vi "Tree Checker.vi"() -> ()   [LabVIEW 2016]
panel:
  in  "Starting at N = ?":i32=2
  out "Finished?":bool
  out "Time By N":cluster{dbl, "Run Time ms":u32}[](graph)
  out "Radio Number By N":cluster{dbl, "Radio Number":i32}[](graph)
  out "Start Value by N":cluster{dbl, "Start Value":i32}[](graph)
  out "Total time Progressed":u32
  in  "Up to N = ?":i32
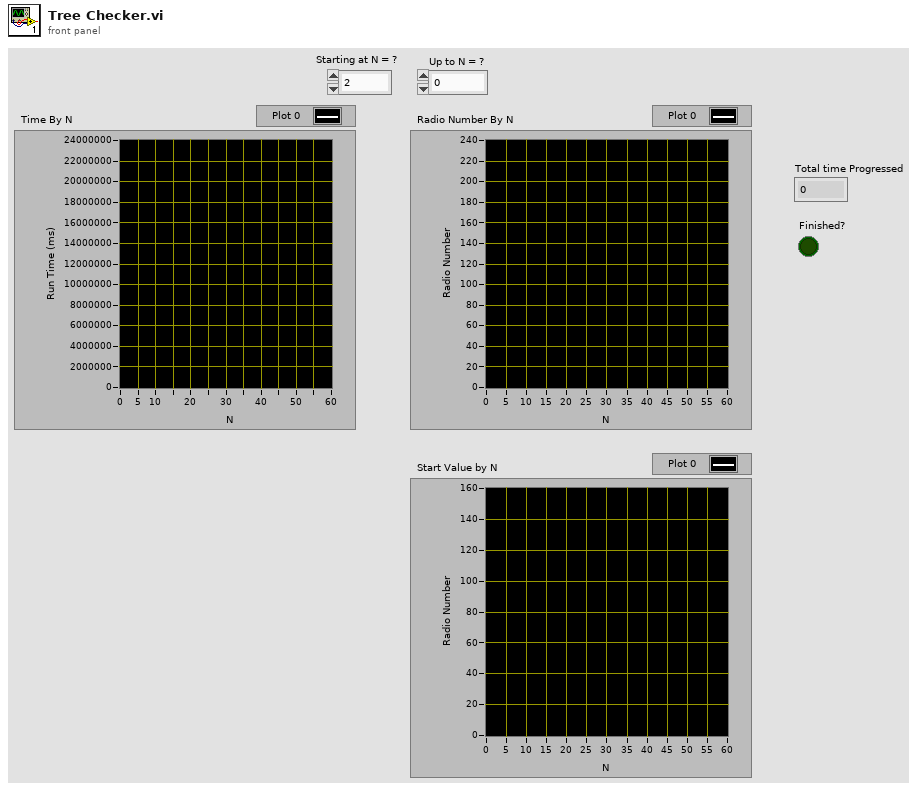
[diagram p1: front panel]
types:
  T1 = typedef "NI_Matrix.lvlib/RealMatrix.ctl" = dbl[][]
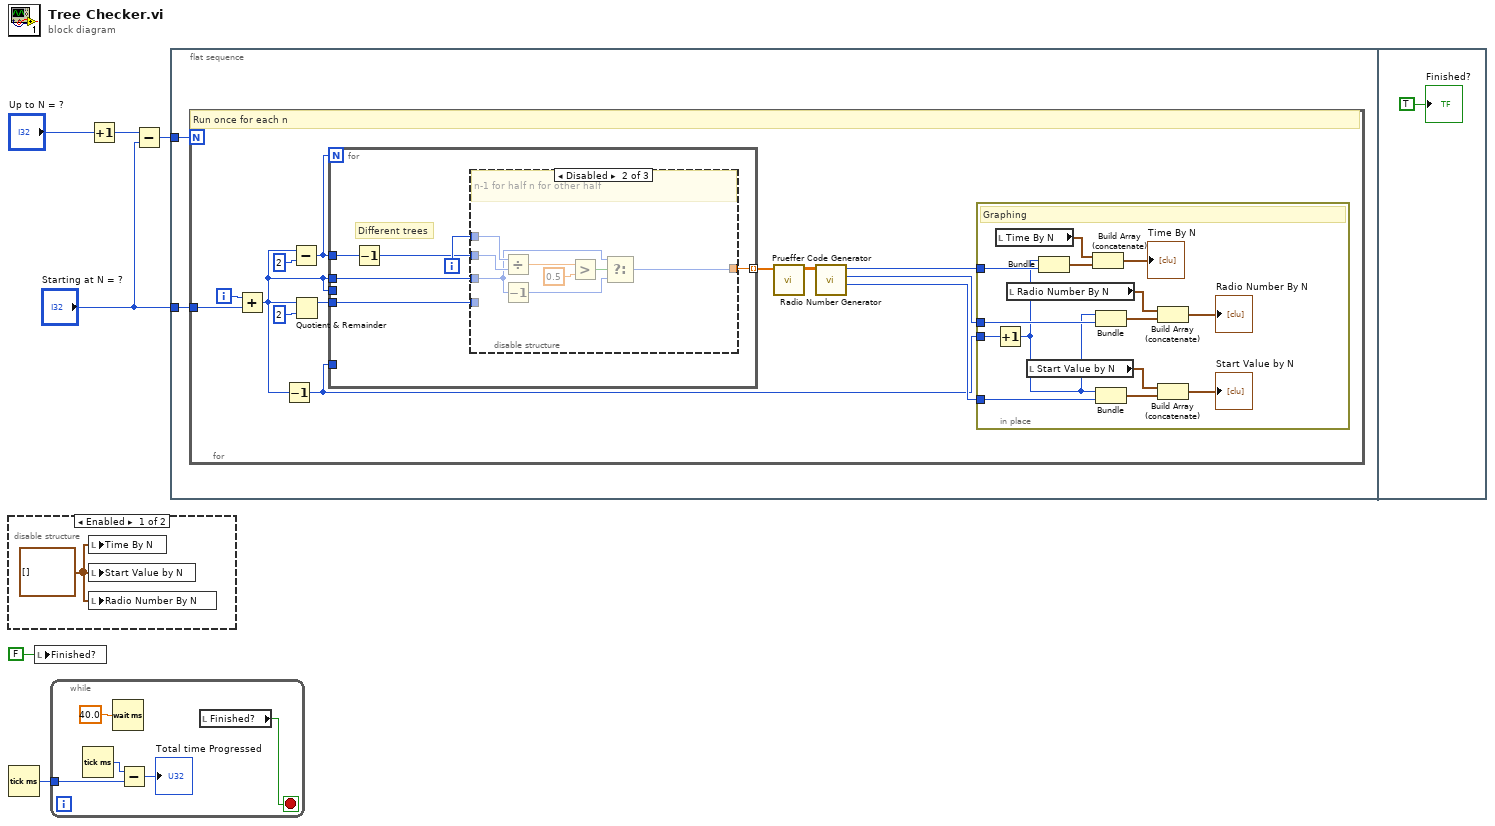
[diagram p0: block diagram]
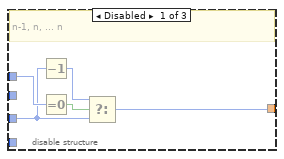
[diagram p2: hidden frame]
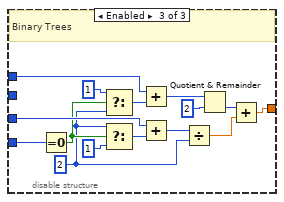
[diagram p3: hidden frame]
diagram:
  n1 = disable-structure shown="Enabled" {
    frame Enabled {
      w7 = cluster{i32, "Radio Number":i32}[] [] ("appended array")
      n2 = local write "Time By N"(w7) -> ()
      n3 = local write "Start Value by N"(w7) -> ()
      n4 = local write "Radio Number By N"(w7) -> ()
    }
    frame Disabled {
    }
  }
  n5 = Tick Count (ms)() -> (millisecond timer value=w4:u32)
  n6 = local write "Finished?"(FALSE) -> ()
  n7 = while {
    tunnel: w4 -> [w9]
    stop <- w11 stop-if-true
    n8 = Tick Count (ms)() -> (millisecond timer value=w10:u32)
    n9 = Wait (ms)(milliseconds to wait=40.0) -> ()  [unwired: 1 out]
    n10 = Subtract(x=w10, y=w9) -> (x-y=→"Total time Progressed":u32)
    n11 = local read "Finished?"() -> (w11:bool)
  }
  n12 = Increment(x="Up to N = ?") -> (x+1=w1:i32)
  n13 = Subtract(x=w1, y="Starting at N = ?") -> (x-y=w5:i32)
  n14 = flat-sequence {
    tunnel: w5 -> [w14]
    tunnel: "Starting at N = ?" -> [w13]
    frame #0 {
      n15 = for {
        N: w14 -> [_]
        tunnel: w13 -> [w24]
        i -> [w27]
        # "Run once for each n"
        n16 = Add(x=w27, y=w24) -> (x+y=w16:i32)
        n17 = Decrement(x=w16) -> (x-1=w19:i32)
        n18 = Subtract(x=w16, y=2) -> (x-y=w18:i32)
        n19 = Quotient & Remainder(x=w16, y=2) -> (x-y*floor(x/y)=w15:i32)  [unwired: 1 out]
        n20 = for {
          N: w18 -> [_]
          tunnel: w16 -> [_]
          tunnel: [w32] -> w22 mode=indexing
          tunnel: w19 -> [_]
          tunnel: w16 -> [w31]
          tunnel: w18 -> [w30]
          tunnel: w15 -> [w28]
          i -> [w33]
          # "Different trees"
          n21 = Decrement(x=w30) -> (x-1=w29:i32)
          n22 = disable-structure shown="Disabled" {
            disable-tunnel: w33 -> [w37 w46 w60]
            disable-tunnel: [w34 w45 w51] -> w32
            disable-tunnel: w31 -> [w36 w39 w55]
            disable-tunnel: w29 -> [_ w44 _]
            disable-tunnel: w28 -> [_ _ w57]
            frame Disabled {
              # "n-1, n, ... n"
              n23 = Decrement(x=w36) -> (x-1=w35:i32)
              n24 = Equal To 0?(x=w37) -> (x = 0?=w38:bool)
              n25 = Select(t=w35, s=w38, f=w36) -> (s? t:f=w34:i32)
            }
            frame Disabled {
              # "n-1 for half n for other half"
              n26 = Divide(x=w46, y=w44) -> (x/y=w43:dbl)
              n27 = Decrement(x=w39) -> (x-1=w40:i32)
              n28 = Greater?(x=w43, y=0.5) -> (0:w41:bool)
              n29 = Select(t=w39, s=w41, f=w40) -> (s? t:f=w45:i32)
            }
            frame Enabled {
              w48 = 2 ("f")
              # "Binary Trees"
              n30 = Equal To 0?(x=w57) -> (x = 0?=w49:bool)
              n31 = Select(t=1 ("y"), s=w49, f=w48) -> (s? t:f=w54:i32)
              n32 = Select(t=w48, s=w49, f=1 ("y")) -> (s? t:f=w47:i32)
              n33 = Add(x=w60, y=w54) -> (x+y=w59:i32)
              n34 = Add(x=w55, y=w47) -> (x+y=w53:i32)
              n35 = Divide(x=w53, y=w48) -> (x/y=w52:dbl)
              n36 = Quotient & Remainder(x=w59, y=2) -> (floor(x/y)=w58:i32)  [unwired: 1 out]
              n37 = Add(x=w58, y=w52) -> (x+y=w51:dbl)
            }
          }
        }
        n38 = call "Prueffer Code Generator.vi"("Array"=w22) -> ("Adjacency Matrix"=w21:T1)  [unwired: 10 in]
        n39 = call "Radio Number Generator.vi"("Adjacency Matrix"=w21) -> ("Start Value"=w23:i32, "Radio Number"=w26:i32, "Run Time ms"=w25:u32)  [unwired: 8 in]
        n40 = in-place {
          in-place-border: w26 -> [w75]
          in-place-border: w25 -> [w74]
          in-place-border: w19 -> [w67]
          in-place-border: w23 -> [w62]
          # "Graphing"
          n41 = Increment(x=w67) -> (x+1=w63:i32)
          n42 = local read "Time By N"() -> (w68:cluster{dbl, "Run Time ms":u32}[])
          n43 = local read "Radio Number By N"() -> (w69:cluster{dbl, "Radio Number":i32}[])
          n44 = local read "Start Value by N"() -> (w66:cluster{dbl, "Start Value":i32}[])
          n45 = Bundle(w63, "Run Time ms"=w74) -> (w73:cluster{i32, "Run Time ms":u32})  [unwired: 1 in]
          n46 = Build Array (concatenate)(w68, w73) -> (→"Time By N":cluster{dbl, "Run Time ms":u32}[])
          n47 = Bundle(w63, "Radio Number"=w75) -> (w71:cluster{i32, "Radio Number":i32})  [unwired: 1 in]
          n48 = Bundle(w63, "Start Value"=w62) -> (w65:cluster{i32, "Start Value":i32})  [unwired: 1 in]
          n49 = Build Array (concatenate)(w69, w71) -> (→"Radio Number By N":cluster{dbl, "Radio Number":i32}[])
          n50 = Build Array (concatenate)(w66, w65) -> (→"Start Value by N":cluster{dbl, "Start Value":i32}[])
        }
      }
    }
    frame #1 {
      "Finished?" <- TRUE
    }
  }
